vi "ReadScanListNode.vi"(8 "Error In":errorcluster, 11 "Multiplexer Node In":refnum<k20>) -> (0 "Error Out":errorcluster, 2 "Scan List":string, 3 "Multiplexer Node Out":refnum<k20>)   [LabVIEW 2012]
uses:
  <vilib>/xml/NI_XML.lvlib
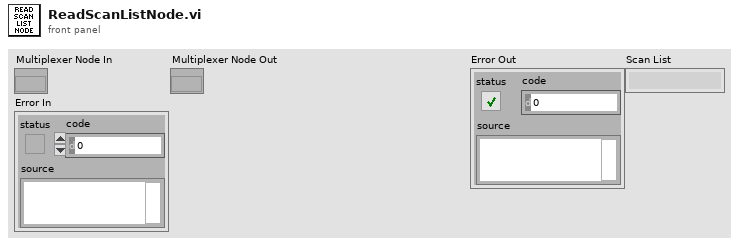
[diagram p1: front panel]
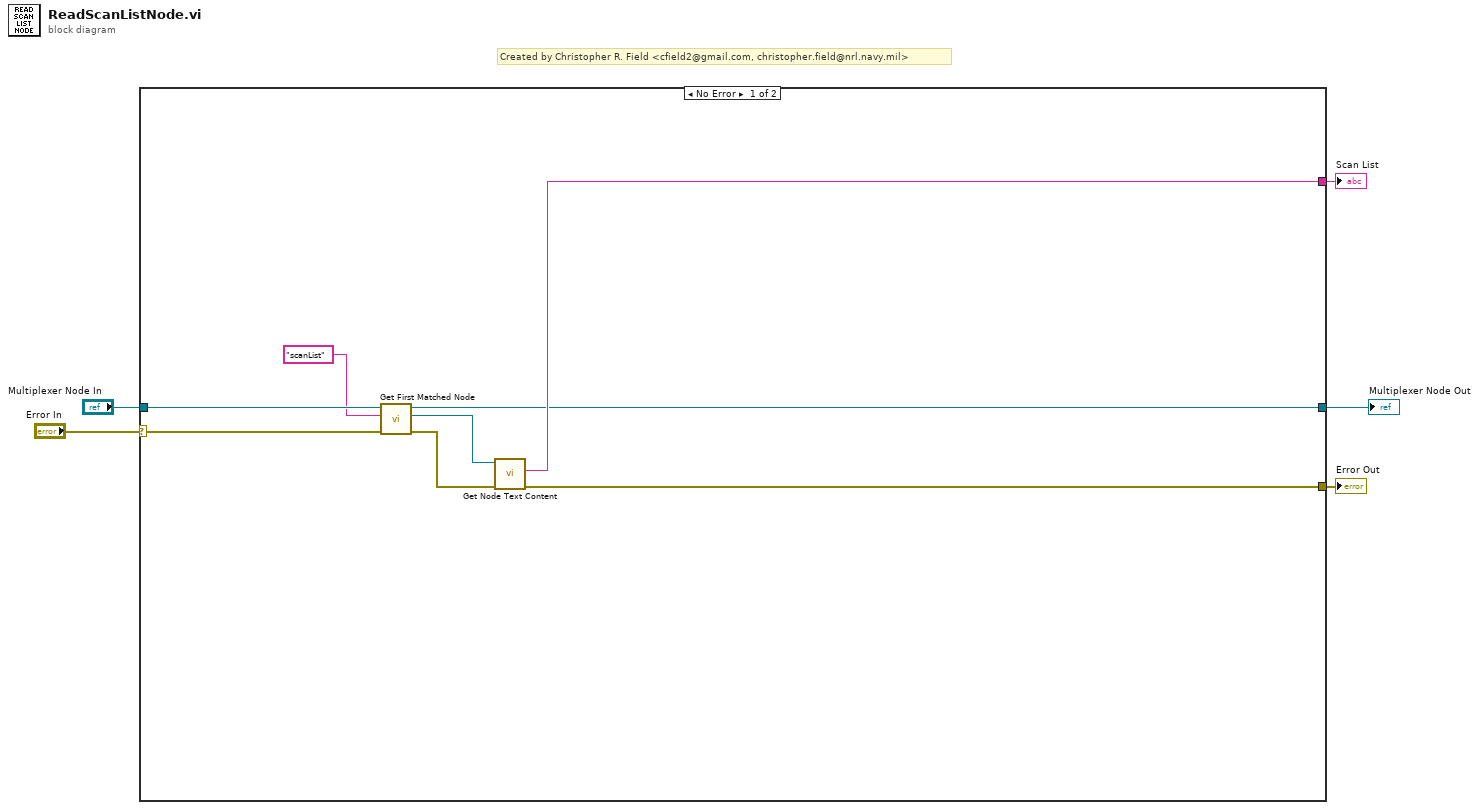
[diagram p0: block diagram]
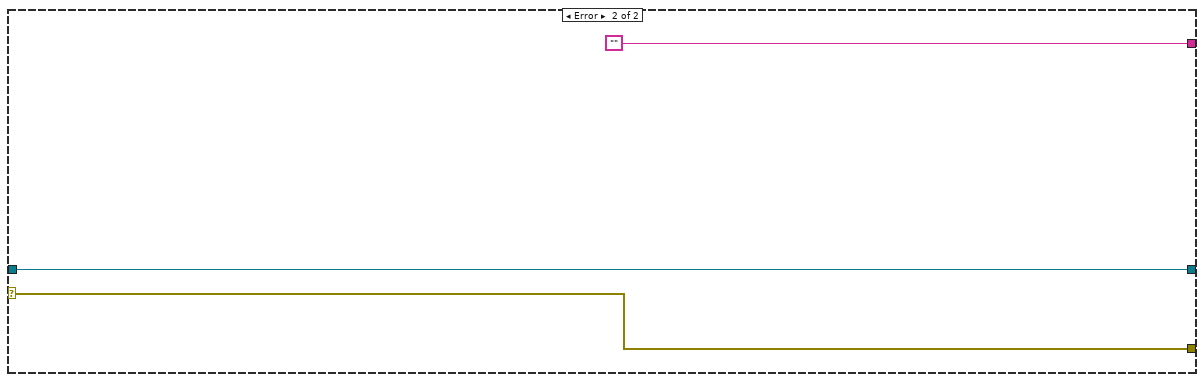
[diagram p2: hidden frame]
diagram:
  # "Created by Christopher R. Field <cfield2@gmail.com, christopher.field@nrl.navy.mil>"
  n1 = case shown="No Error" "Error In" {
    selector: "Error In" -> [w12 w15]
    tunnel: "Multiplexer Node In" -> [w13 w16]
    tunnel: [w8 w15] -> w3
    tunnel: [w7 ""] -> w2
    tunnel: [w6 w16] -> w1
    frame No Error {
      n2 = call <vilib>:"Get First Matched Node.vi"("error in (no error)"=w12, "XPath expression"="scanList", "node in"=w13) -> ("error out"=w9:errorcluster, "node result"=w10:refnum<k20>, "node out"=w6:refnum<k20>)  [unwired: 6 in]
      n3 = call <vilib>:"Get Node Text Content.vi"("error in (no error)"=w9, "node in"=w10) -> ("error out"=w8:errorcluster, "node text"=w7:string)  [unwired: 7 in, 1 out]
    }
    frame Error {
    }
  }
  "Error Out" <- w3
  "Scan List" <- w2
  "Multiplexer Node Out" <- w1
